vi "chart series set name lv.vi"(8 "error in (no error)":errorcluster, 10 "name":string, 11 "series":u32) -> (0 "error out":errorcluster)   [LabVIEW 2015, in "xlsxwriter.lvlib"]
doc: "void chart_series_set_name_lv(lxw_chart_series series, const char *name);"
uses:
  xlsxwriter.lvlib
  xlsxwriter.dll
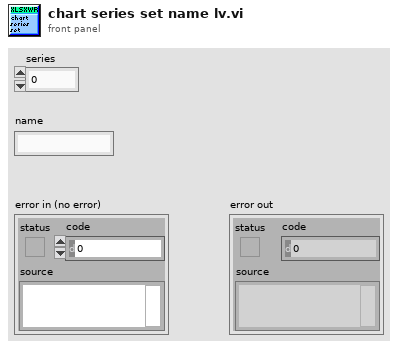
[diagram p1: front panel]
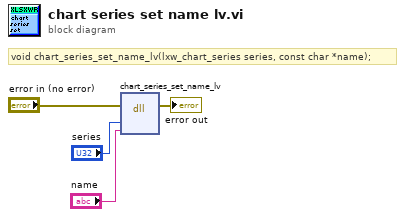
[diagram p0: block diagram]
diagram:
  # "void chart_series_set_name_lv(lxw_chart_series series, const char *name);"
  n1 = dll-call lib="C:/Users/WDAGUtilityAccount/Desktop/lv_vis_added_cell/xlsxwriter.*" fn="chart_series_set_name_lv"(error in="error in (no error)", "series"="series", "name"="name") -> (error out=→"error out":errorcluster)  [unwired: 5 in, 1 out]
